vi "DSF.Engine.Transceiver Thread.Transfer Group.Get by ID.vi"(8 "error in (no error)":errorcluster, 10 "Transfer Group id":i32, 11 "Transceiver Thread in":refnum<class "DSF.Engine.Transceiver Thread.lvclass">) -> (0 "error out":errorcluster, 2 "Transfer Group":refnum<class "DSF.Engine.Transfer Group.lvclass">, 3 "Transceiver Thread out":refnum<class "DSF.Engine.Transceiver Thread.lvclass">)   [LabVIEW 2017, in "DSF.Engine.lvlib" / "DSF.Engine.Transceiver Thread.lvclass"]
uses:
  DSF.Engine.Transceiver Thread.lvclass
  Transfer/DSF.Engine.Transfer Group.lvclass
  DSF.Engine.Transceiver Thread.lvclass/DSF.Engine.Transceiver Thread.ctl
  Cache/DSF.Engine.Memory.Cache.lvclass/DSF.Engine.Memory.Cache.ctl
  Cache/DSF.Engine.Memory.Cache.Get Transfers Groups.vi
  Cache/DSF.Engine.Memory.Cache.lvclass
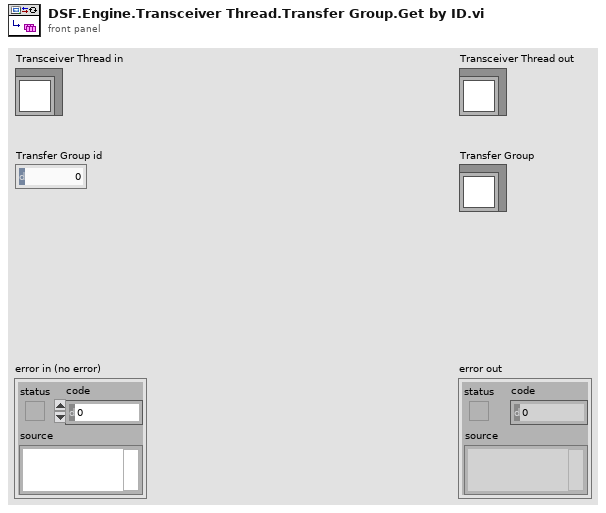
[diagram p1: front panel]
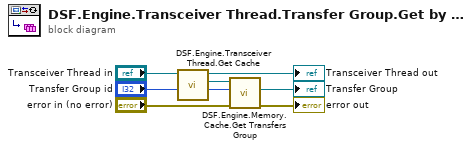
[diagram p0: block diagram]
diagram:
  n1 = call "DSF.Engine.Transceiver Thread.Get Cache.vi"("Transceiver Thread in"="Transceiver Thread in") -> ("Cache"=w3:refnum<class "DSF.Engine.Memory.Cache.lvclass">, "Transceiver Thread out"=→"Transceiver Thread out":refnum<class "DSF.Engine.Transceiver Thread.lvclass">)  [unwired: 9 in]
  n2 = call "DSF.Engine.Memory.Cache.Get Transfers Group.vi"("Transfer Group id"="Transfer Group id", "Cache in"=w3) -> ("Transfers Group"=→"Transfer Group":refnum<class "DSF.Engine.Transfer Group.lvclass">)  [unwired: 8 in, 1 out]
  "error out" <- "error in (no error)"
